vi "SP_OEE_2_test.vi"() -> ()   [LabVIEW 2017] (continued)
                      tunnel: [w1109] -> w922
                      tunnel: w1000 -> [w1148]
                      tunnel: w999 -> [w1147]
                      tunnel: w998 -> [w1146]
                      tunnel: w997 -> [w1142]
                      tunnel: w996 -> [w1145]
                      tunnel: w995 -> [w1144]
                      tunnel: w994 -> [w1140]
                      tunnel: w993 -> [w1138]
                      tunnel: w992 -> [w1137]
                      tunnel: [w1148] -> w988
                      tunnel: [w1147] -> w987
                      tunnel: [w1146] -> w986
                      tunnel: [w1145] -> w985
                      tunnel: [w1144] -> w984
                      tunnel: [w1141] -> w983
                      tunnel: [w1135] -> w982
                      tunnel: [w1134] -> w981
                      tunnel: [w1139] -> w980
                      tunnel: [w1138] -> w979
                      tunnel: [w1137] -> w978
                      tunnel: w991 -> [w1133]
                      tunnel: [w1133] -> w977
                      tunnel: w990 -> [w1130]
                      tunnel: [w1130] -> w976
                      tunnel: [w1129] -> w975
                      tunnel: w989 -> [w1129]
                      tunnel: w922 -> [w1128]
                      tunnel: [w1128] -> w921
                      tunnel: w988 -> [w1171]
                      tunnel: w987 -> [w1170]
                      tunnel: w986 -> [w1169]
                      tunnel: w985 -> [w1168]
                      tunnel: w984 -> [w1167]
                      tunnel: w983 -> [w1163]
                      tunnel: w982 -> [w1166]
                      tunnel: w981 -> [w1165]
                      tunnel: w980 -> [w1162]
                      tunnel: w979 -> [w1159]
                      tunnel: w978 -> [w1158]
                      tunnel: [w1171] -> w974
                      tunnel: [w1170] -> w973
                      tunnel: [w1169] -> w972
                      tunnel: [w1168] -> w971
                      tunnel: [w1167] -> w970
                      tunnel: [w1166] -> w969
                      tunnel: [w1165] -> w968
                      tunnel: [w1161] -> w967
                      tunnel: [w1160] -> w966
                      tunnel: [w1156] -> w965
                      tunnel: [w1155] -> w964
                      tunnel: [w1159] -> w963
                      tunnel: [w1158] -> w962
                      tunnel: w977 -> [w1154]
                      tunnel: [w1154] -> w961
                      tunnel: w976 -> [w1151]
                      tunnel: [w1151] -> w960
                      tunnel: [w1150] -> w959
                      tunnel: w975 -> [w1150]
                      tunnel: w921 -> [w1149]
                      tunnel: [w1149] -> w920
                      tunnel: w974 -> [w1196]
                      tunnel: w973 -> [w1195]
                      tunnel: w972 -> [w1194]
                      tunnel: w971 -> [w1193]
                      tunnel: w970 -> [w1192]
                      tunnel: w969 -> [w1191]
                      tunnel: w968 -> [w1190]
                      tunnel: w967 -> [w1184]
                      tunnel: w966 -> [w1186]
                      tunnel: w965 -> [w1189]
                      tunnel: w964 -> [w1188]
                      tunnel: w963 -> [w1181]
                      tunnel: w962 -> [w1182]
                      tunnel: [w1196] -> w958
                      tunnel: [w1195] -> w957
                      tunnel: [w1194] -> w956
                      tunnel: [w1193] -> w955
                      tunnel: [w1192] -> w954
                      tunnel: [w1191] -> w953
                      tunnel: [w1190] -> w952
                      tunnel: [w1189] -> w951
                      tunnel: [w1188] -> w950
                      tunnel: [w1185] -> w949
                      tunnel: [w1183] -> w948
                      tunnel: [w1179] -> w947
                      tunnel: [w1177] -> w946
                      tunnel: w961 -> [w1178]
                      tunnel: w960 -> [w1174]
                      tunnel: [w1173] -> w945
                      tunnel: w959 -> [w1173]
                      tunnel: w920 -> [w1172]
                      tunnel: w958 -> [w1223]
                      tunnel: w957 -> [w1216]
                      tunnel: w956 -> [w1207]
                      tunnel: w955 -> [w1215]
                      tunnel: w954 -> [w1205]
                      tunnel: w953 -> [w1214]
                      tunnel: w952 -> [w1203]
                      tunnel: w951 -> [w1213]
                      tunnel: w950 -> [w1201]
                      tunnel: w949 -> [w1237]
                      tunnel: w948 -> [w1236]
                      tunnel: w947 -> [w1212]
                      tunnel: w946 -> [w1199]
                      tunnel: [w1237] -> w944
                      tunnel: [w1236] -> w943
                      tunnel: [w1230] -> w942
                      tunnel: [w1223] -> w941
                      tunnel: [w1222] -> w940
                      tunnel: [w1221] -> w939
                      tunnel: [w1220] -> w938
                      tunnel: [w1219] -> w937
                      tunnel: [w1218] -> w936
                      tunnel: [w1217] -> w935
                      tunnel: [w1216] -> w934
                      tunnel: [w1215] -> w933
                      tunnel: [w1214] -> w932
                      tunnel: [w1213] -> w931
                      tunnel: [w1212] -> w930
                      tunnel: [w1197] -> w929
                      tunnel: w945 -> [w1197]
                      tunnel: [w1257] -> w904
                      tunnel: [w1243] -> w902
                      tunnel: w944 -> [w1244]
                      tunnel: w943 -> [w1257]
                      tunnel: w942 -> [w1242]
                      tunnel: w941 -> [w1255]
                      tunnel: w940 -> [w1253]
                      tunnel: w939 -> [w1251]
                      tunnel: w938 -> [w1249]
                      tunnel: w937 -> [w1247]
                      tunnel: w936 -> [w1245]
                      tunnel: w935 -> [w1238]
                      tunnel: w934 -> [w1254]
                      tunnel: w933 -> [w1252]
                      tunnel: w932 -> [w1250]
                      tunnel: w931 -> [w1248]
                      tunnel: w930 -> [w1246]
                      tunnel: w929 -> [w1241]
                      tunnel: [w1238] -> w916
                      frame #0 {
                        w1033 = "%Y-%m-%d" ("time format string (%c)")
                        n185 = Decimal String To Number(string=w1020) -> (number=w1019:i32)  [unwired: 2 in, 1 out]
                        n186 = property on="Table" class="Tbl (strict)"("Visible"=TRUE) -> ()  [unwired: 2 in, 2 out]
                        n187 = Format Date/Time String(time format string (%c)=w1033, seconds (now)=w1025) -> (date/time string=w1034:string)  [unwired: 1 in]
                        n188 = Format Date/Time String(time format string (%c)=w1033, seconds (now)=w1024) -> (date/time string=w1032:string)  [unwired: 1 in]
                        n189 = Format Into String(format string="Where BREAKDOWN_DATE between '%s' and '%s' and  SHIFT_ID = '%d'  ", w1034, w1032, w1019) -> (resulting string=w1031:string)  [unwired: 2 in, 1 out]
                        n190 = call <vilib>:"DB Tools Select Data.vi"("condition"=w1031, "error in (no error)"=w1040, "columns"=string[] ["BREAKDOWN_DATE"], "table"="STATION_1_LOG_HISTORY", "connection reference"=w1042) -> ("error out"=w1027:errorcluster, "data"=w1030:variant[][], "connection reference out"=w1041:T2)  [unwired: 1 in]
                        n191 = property on="Table 2" class="Tbl (strict)"("Visible"=FALSE) -> ()  [unwired: 2 in, 2 out]
                        n192 = xnode "Database Variant To Data"("database variant"=w1030, "error in (no error)"=w1027, "type"=string[][] [] ("Elements Found")) -> ("data"=w1028:string[][], "error out"=w1026:errorcluster)
                        n193 = Index Array(array=w1028, index (col)=0 ("disabled index (col)")) -> (element=w1036:string[])  [unwired: 1 in]
                        n194 = call "Search_1d_array_element.vi"("Count in"=string[] [] ("Elements Found"), "BD Date"=w1036, "Elements Found in"=string[] [] ("Elements Found")) -> ("Elements Found out"=w1022:string[])  [unwired: 4 in, 2 out]
                        n195 = Build Array(w1022) -> (w1046:string[][])
                        n196 = Transpose 2D Array(2D array=w1046) -> (transposed array=w1045:string[][])
                      }
                      frame #1 {
                        n197 = call "Stack_holderwise_total_bd_count_&_duration_2.vi"("Refnum in"=w1108, "BREAKDOWN_STK_HOLD_ID"=1, "condition"=w1095, "Form Date"=w1102, "To Date"=w1101, "error in (no error)"=w1106, "Shift"=w1092) -> ("Refnum out"=w1107:T2, "Count out"=w1100:string[], "appended array"=w1097:dbl[], "error out"=w1105:errorcluster)  [unwired: 5 in]
                        n198 = call "NUMERIC TO STRING.vi"("appended array"=w1097) -> ("Array"=w1096:string[])  [unwired: 4 in]
                        n199 = call "Insert_empty_element_with_zero.vi"("searched date"=w1100, "fixed date"=w1098) -> ("O/P"=w1093:string[])  [unwired: 9 in]
                        n200 = call "Insert_empty_element_with_zero.vi"("searched date"=w1096, "fixed date"=w1098) -> ("O/P"=w1099:string[])  [unwired: 9 in]
                      }
                      frame #2 {
                        n201 = call "Stack_holderwise_total_bd_count_&_duration_2.vi"("Refnum in"=w1122, "BREAKDOWN_STK_HOLD_ID"=2, "condition"=w1111, "Form Date"=w1119, "To Date"=w1118, "error in (no error)"=w1124, "Shift"=w1109) -> ("Refnum out"=w1120:T2, "Count out"=w1117:string[], "appended array"=w1113:dbl[], "error out"=w1123:errorcluster)  [unwired: 5 in]
                        n202 = call "Insert_empty_element_with_zero.vi"("searched date"=w1117, "fixed date"=w1114) -> ("O/P"=w1116:string[])  [unwired: 9 in]
                        n203 = call "NUMERIC TO STRING.vi"("appended array"=w1113) -> ("Array"=w1112:string[])  [unwired: 4 in]
                        n204 = call "Insert_empty_element_with_zero.vi"("searched date"=w1112, "fixed date"=w1114) -> ("O/P"=w1115:string[])  [unwired: 9 in]
                      }
                      frame #3 {
                        n205 = call "Stack_holderwise_total_bd_count_&_duration_2.vi"("Refnum in"=w1140, "BREAKDOWN_STK_HOLD_ID"=3, "condition"=w1130, "Form Date"=w1138, "To Date"=w1137, "error in (no error)"=w1142, "Shift"=w1128) -> ("Refnum out"=w1139:T2, "Count out"=w1136:string[], "appended array"=w1132:dbl[], "error out"=w1141:errorcluster)  [unwired: 5 in]
                        n206 = call "Insert_empty_element_with_zero.vi"("searched date"=w1136, "fixed date"=w1133) -> ("O/P"=w1135:string[])  [unwired: 9 in]
                        n207 = call "NUMERIC TO STRING.vi"("appended array"=w1132) -> ("Array"=w1131:string[])  [unwired: 4 in]
                        n208 = call "Insert_empty_element_with_zero.vi"("searched date"=w1131, "fixed date"=w1133) -> ("O/P"=w1134:string[])  [unwired: 9 in]
                      }
                      frame #4 {
                        n209 = call "Stack_holderwise_total_bd_count_&_duration_2.vi"("Refnum in"=w1162, "BREAKDOWN_STK_HOLD_ID"=4, "condition"=w1151, "Form Date"=w1159, "To Date"=w1158, "error in (no error)"=w1163, "Shift"=w1149) -> ("Refnum out"=w1161:T2, "Count out"=w1157:string[], "appended array"=w1153:dbl[], "error out"=w1160:errorcluster)  [unwired: 5 in]
                        n210 = call "Insert_empty_element_with_zero.vi"("searched date"=w1157, "fixed date"=w1154) -> ("O/P"=w1156:string[])  [unwired: 9 in]
                        n211 = call "NUMERIC TO STRING.vi"("appended array"=w1153) -> ("Array"=w1152:string[])  [unwired: 4 in]
                        n212 = call "Insert_empty_element_with_zero.vi"("searched date"=w1152, "fixed date"=w1154) -> ("O/P"=w1155:string[])  [unwired: 9 in]
                      }
                      frame #5 {
                        n213 = call "Stack_holderwise_total_bd_count_&_duration_2.vi"("Refnum in"=w1184, "BREAKDOWN_STK_HOLD_ID"=5, "condition"=w1174, "Form Date"=w1181, "To Date"=w1182, "error in (no error)"=w1186, "Shift"=w1172) -> ("Refnum out"=w1183:T2, "Count out"=w1180:string[], "appended array"=w1176:dbl[], "error out"=w1185:errorcluster)  [unwired: 5 in]
                        n214 = call "NUMERIC TO STRING.vi"("appended array"=w1176) -> ("Array"=w1175:string[])  [unwired: 4 in]
                        n215 = call "Insert_empty_element_with_zero.vi"("searched date"=w1180, "fixed date"=w1178) -> ("O/P"=w1179:string[])  [unwired: 9 in]
                        n216 = call "Insert_empty_element_with_zero.vi"("searched date"=w1175, "fixed date"=w1178) -> ("O/P"=w1177:string[])  [unwired: 9 in]
                      }
                      frame #6 {
                        n217 = call "String to numeric.vi"("Array"=w1207) -> ("Array 2"=w1206:dbl[])  [unwired: 4 in]
                        n218 = call "String to numeric.vi"("Array"=w1205) -> ("Array 2"=w1204:dbl[])  [unwired: 4 in]
                        n219 = call "String to numeric.vi"("Array"=w1203) -> ("Array 2"=w1202:dbl[])  [unwired: 4 in]
                        n220 = call "String to numeric.vi"("Array"=w1201) -> ("Array 2"=w1200:dbl[])  [unwired: 4 in]
                        n221 = call "String to numeric.vi"("Array"=w1199) -> ("Array 2"=w1198:dbl[])  [unwired: 4 in]
                        n222 = Decimal String To Number(string=w1212) -> (number=w1231:i32[])  [unwired: 2 in, 1 out]
                        n223 = Decimal String To Number(string=w1213) -> (number=w1232:i32[])  [unwired: 2 in, 1 out]
                        n224 = Decimal String To Number(string=w1214) -> (number=w1233:i32[])  [unwired: 2 in, 1 out]
                        n225 = Decimal String To Number(string=w1215) -> (number=w1234:i32[])  [unwired: 2 in, 1 out]
                        n226 = Decimal String To Number(string=w1216) -> (number=w1229:i32[])  [unwired: 2 in, 1 out]
                        n227 = Compound Arithmetic op=ADD(w1206, w1204, w1202, w1200, w1198) -> (w1209:dbl[])
                        n228 = Build Array(w1207) -> (w1228:string[][])
                        n229 = Build Array(w1205) -> (w1227:string[][])
                        n230 = Build Array(w1203) -> (w1226:string[][])
                        n231 = Build Array(w1201) -> (w1225:string[][])
                        n232 = Build Array(w1199) -> (w1224:string[][])
                        n233 = Number To Fractional String(number=w1209, precision (6)=i16 2) -> (F-format string=w1208:string[])  [unwired: 2 in]
                        n234 = Compound Arithmetic op=ADD(w1231, w1232, w1233, w1234, w1229) -> (w1235:i32[])
                        n235 = Transpose 2D Array(2D array=w1228) -> (transposed array=w1222:string[][])
                        n236 = Transpose 2D Array(2D array=w1227) -> (transposed array=w1221:string[][])
                        n237 = Transpose 2D Array(2D array=w1226) -> (transposed array=w1220:string[][])
                        n238 = Transpose 2D Array(2D array=w1225) -> (transposed array=w1219:string[][])
                        n239 = Transpose 2D Array(2D array=w1224) -> (transposed array=w1218:string[][])
                        n240 = Number To Decimal String(number=w1235) -> (decimal integer string=w1230:string[])  [unwired: 1 in]
                        n241 = Build Array(w1208) -> (w1211:string[][])
                        n242 = Transpose 2D Array(2D array=w1211) -> (transposed array=w1217:string[][])
                      }
                      frame #7 {
                        n243 = Insert Into Array(array=w1255, index (col)=1 ("disabled index (col)"), new element #1=w1254, new element #2=w1253, new element #3=w1252, new element #4=w1251, new element #5=w1250, new element #6=w1249, new element #7=w1248, new element #8=w1247, new element #9=w1246, new element #10=w1245, new element #11=w1242, new element #12=w1238) -> (w1240:string[][])  [unwired: 1 in]
                        n244 = call "flot graph for month n year.vi"("BD Date"=w1241, "error in (no error)"=w1244, "Count total"=w1242) -> ("error out"=w1243:errorcluster, "Run-Time Status"=w1239:cluster{"Array 2":timestamp[], dbl[]})  [unwired: 7 in]
                        n245 = local write "Run-Time Status"(w1239) -> ()
                        n246 = local write "Table"(w1240) -> ()
                      }
                    }
                    n247 = call "OEE_PART_1.vi"("CYCLE TIME"=w917, "ACTUAL PROD TIME"=w918, "BREAKDOWN TOTAL TIME"=w916) -> ("Numeric"=w907:i32, "CAPACITY"=w905:dbl, "ACTUAL TIME"=w906:i32)  [unwired: 5 in, 1 out]
                    n248 = call "OEE_PART_2_P.vi"("Refnum in"=w904, "Shift"=w913, "String"="ALL", "Select Station"=w911, "Form Date"=w915, "To Date"=w914, "AVAILABLILITY TIME"=w906, "CAPACITY"=w905) -> ("Refnum out"=w903:T2, "QUALITY"=w910:dbl, "OEE"=w908:dbl, "PERFORMANCE"=w909:dbl)  [unwired: 2 in, 2 out]
                    n249 = local write "PERFORMANCE"(w909) -> ()
                    n250 = local write "QUALITY"(w910) -> ()
                    n251 = local write "OEE"(w908) -> ()
                    n252 = local write "AVAILABLILITY TIME(MIN)"(w906) -> ()
                    n253 = local write "IDEAL CYCLE TIME"(w907) -> ()
                    n254 = local write "CAPACITY"(w905) -> ()
                  }
                  frame "3" {
                    n255 = flat-sequence {
                      tunnel: w1284 -> [w1398]
                      tunnel: w1283 -> [w1396]
                      tunnel: [w1382] -> w1374
                      tunnel: [w1397] -> w1373
                      tunnel: w1282 -> [_]
                      tunnel: [w1401] -> w1372
                      tunnel: [w1381] -> w1371
                      tunnel: [w1380] -> w1370
                      tunnel: [w1378] -> w1369
                      tunnel: w1281 -> [w1381]
                      tunnel: w1280 -> [w1380]
                      tunnel: ["Where BREAKDOWN_DATE between '%s'and '%s' and BREAKDOWN_STK_HOLD_ID ='%d' and  SHIFT_ID = '%d' "] -> w1368
                      tunnel: [w1378] -> w1367
                      tunnel: w1275 -> [w1376]
                      tunnel: w1374 -> [w1462]
                      tunnel: w1373 -> [w1464]
                      tunnel: w1372 -> [w1459]
                      tunnel: w1371 -> [w1458]
                      tunnel: w1370 -> [w1457]
                      tunnel: [w1461] -> w1366
                      tunnel: [w1463] -> w1365
                      tunnel: [w1459] -> w1364
                      tunnel: [w1449] -> w1363
                      tunnel: [w1455] -> w1362
                      tunnel: [w1458] -> w1361
                      tunnel: [w1457] -> w1360
                      tunnel: w1369 -> [w1454]
                      tunnel: [w1454] -> w1359
                      tunnel: w1368 -> [w1451]
                      tunnel: [w1451] -> w1358
                      tunnel: [w1450] -> w1357
                      tunnel: w1367 -> [w1450]
                      tunnel: w1275 -> [w1448]
                      tunnel: [w1448] -> w1279
                      tunnel: w1366 -> [w1480]
                      tunnel: w1365 -> [w1478]
                      tunnel: w1364 -> [w1483]
                      tunnel: w1363 -> [w1482]
                      tunnel: w1362 -> [w1481]
                      tunnel: w1361 -> [w1475]
                      tunnel: w1360 -> [w1474]
                      tunnel: [w1483] -> w1356
                      tunnel: [w1482] -> w1355
                      tunnel: [w1481] -> w1354
                      tunnel: [w1479] -> w1353
                      tunnel: [w1472] -> w1352
                      tunnel: [w1471] -> w1351
                      tunnel: [w1476] -> w1350
                      tunnel: [w1475] -> w1349
                      tunnel: [w1474] -> w1348
                      tunnel: w1359 -> [w1470]
                      tunnel: [w1470] -> w1347
                      tunnel: w1358 -> [w1467]
                      tunnel: [w1467] -> w1346
                      tunnel: [w1466] -> w1345
                      tunnel: w1357 -> [w1466]
                      tunnel: w1279 -> [w1465]
                      tunnel: [w1465] -> w1278
                      tunnel: w1356 -> [w1504]
                      tunnel: w1355 -> [w1503]
                      tunnel: w1354 -> [w1502]
                      tunnel: w1353 -> [w1498]
                      tunnel: w1352 -> [w1501]
                      tunnel: w1351 -> [w1500]
                      tunnel: w1350 -> [w1496]
                      tunnel: w1349 -> [w1494]
                      tunnel: w1348 -> [w1493]
                      tunnel: [w1504] -> w1344
                      tunnel: [w1503] -> w1343
                      tunnel: [w1502] -> w1342
                      tunnel: [w1501] -> w1341
                      tunnel: [w1500] -> w1340
                      tunnel: [w1497] -> w1339
                      tunnel: [w1491] -> w1338
                      tunnel: [w1490] -> w1337
                      tunnel: [w1495] -> w1336
                      tunnel: [w1494] -> w1335
                      tunnel: [w1493] -> w1334
                      tunnel: w1347 -> [w1489]
                      tunnel: [w1489] -> w1333
                      tunnel: w1346 -> [w1486]
                      tunnel: [w1486] -> w1332
                      tunnel: [w1485] -> w1331
                      tunnel: w1345 -> [w1485]
                      tunnel: w1278 -> [w1484]
                      tunnel: [w1484] -> w1277
                      tunnel: w1344 -> [w1527]
                      tunnel: w1343 -> [w1526]
                      tunnel: w1342 -> [w1525]
                      tunnel: w1341 -> [w1524]
                      tunnel: w1340 -> [w1523]
                      tunnel: w1339 -> [w1519]
                      tunnel: w1338 -> [w1522]
                      tunnel: w1337 -> [w1521]
                      tunnel: w1336 -> [w1518]
                      tunnel: w1335 -> [w1515]
                      tunnel: w1334 -> [w1514]
                      tunnel: [w1527] -> w1330
                      tunnel: [w1526] -> w1329
                      tunnel: [w1525] -> w1328
                      tunnel: [w1524] -> w1327
                      tunnel: [w1523] -> w1326
                      tunnel: [w1522] -> w1325
                      tunnel: [w1521] -> w1324
                      tunnel: [w1517] -> w1323
                      tunnel: [w1516] -> w1322
                      tunnel: [w1512] -> w1321
                      tunnel: [w1511] -> w1320
                      tunnel: [w1515] -> w1319
                      tunnel: [w1514] -> w1318
                      tunnel: w1333 -> [w1510]
                      tunnel: [w1510] -> w1317
                      tunnel: w1332 -> [w1507]
                      tunnel: [w1507] -> w1316
                      tunnel: [w1506] -> w1315
                      tunnel: w1331 -> [w1506]
                      tunnel: w1277 -> [w1505]
                      tunnel: [w1505] -> w1276
                      tunnel: w1330 -> [w1552]
                      tunnel: w1329 -> [w1551]
                      tunnel: w1328 -> [w1550]
                      tunnel: w1327 -> [w1549]
                      tunnel: w1326 -> [w1548]
                      tunnel: w1325 -> [w1547]
                      tunnel: w1324 -> [w1546]
                      tunnel: w1323 -> [w1540]
                      tunnel: w1322 -> [w1542]
                      tunnel: w1321 -> [w1545]
                      tunnel: w1320 -> [w1544]
                      tunnel: w1319 -> [w1537]
                      tunnel: w1318 -> [w1538]
                      tunnel: [w1552] -> w1314
                      tunnel: [w1551] -> w1313
                      tunnel: [w1550] -> w1312
                      tunnel: [w1549] -> w1311
                      tunnel: [w1548] -> w1310
                      tunnel: [w1547] -> w1309
                      tunnel: [w1546] -> w1308
                      tunnel: [w1545] -> w1307
                      tunnel: [w1544] -> w1306
                      tunnel: [w1541] -> w1305
                      tunnel: [w1539] -> w1304
                      tunnel: [w1535] -> w1303
                      tunnel: [w1533] -> w1302
                      tunnel: w1317 -> [w1534]
                      tunnel: w1316 -> [w1530]
                      tunnel: [w1529] -> w1301
                      tunnel: w1315 -> [w1529]
                      tunnel: w1276 -> [w1528]
                      tunnel: w1314 -> [w1579]
                      tunnel: w1313 -> [w1572]
                      tunnel: w1312 -> [w1563]
                      tunnel: w1311 -> [w1571]
                      tunnel: w1310 -> [w1561]
                      tunnel: w1309 -> [w1570]
                      tunnel: w1308 -> [w1559]
                      tunnel: w1307 -> [w1569]
                      tunnel: w1306 -> [w1557]
                      tunnel: w1305 -> [w1593]
                      tunnel: w1304 -> [w1592]
                      tunnel: w1303 -> [w1568]
                      tunnel: w1302 -> [w1555]
                      tunnel: [w1593] -> w1300
                      tunnel: [w1592] -> w1299
                      tunnel: [w1586] -> w1298
                      tunnel: [w1579] -> w1297
                      tunnel: [w1578] -> w1296
                      tunnel: [w1577] -> w1295
                      tunnel: [w1576] -> w1294
                      tunnel: [w1575] -> w1293
                      tunnel: [w1574] -> w1292
                      tunnel: [w1573] -> w1291
                      tunnel: [w1572] -> w1290
                      tunnel: [w1571] -> w1289
                      tunnel: [w1570] -> w1288
                      tunnel: [w1569] -> w1287
                      tunnel: [w1568] -> w1286
                      tunnel: [w1553] -> w1285
                      tunnel: w1301 -> [w1553]
                      tunnel: [w1613] -> w1260
                      tunnel: [w1599] -> w1258
                      tunnel: w1300 -> [w1600]
                      tunnel: w1299 -> [w1613]
                      tunnel: w1298 -> [w1598]
                      tunnel: w1297 -> [w1611]
                      tunnel: w1296 -> [w1609]
                      tunnel: w1295 -> [w1607]
                      tunnel: w1294 -> [w1605]
                      tunnel: w1293 -> [w1603]
                      tunnel: w1292 -> [w1601]
                      tunnel: w1291 -> [w1594]
                      tunnel: w1290 -> [w1610]
                      tunnel: w1289 -> [w1608]
                      tunnel: w1288 -> [w1606]
                      tunnel: w1287 -> [w1604]
                      tunnel: w1286 -> [w1602]
                      tunnel: w1285 -> [w1597]
                      tunnel: [w1594] -> w1271
                      frame #0 {
                        w1389 = "%Y-%m-%d" ("time format string (%c)")
                        n256 = Decimal String To Number(string=w1376) -> (number=w1375:i32)  [unwired: 2 in, 1 out]
                        n257 = property on="Table" class="Tbl (strict)"("Visible"=TRUE) -> ()  [unwired: 2 in, 2 out]
                        n258 = Format Date/Time String(time format string (%c)=w1389, seconds (now)=w1381) -> (date/time string=w1390:string)  [unwired: 1 in]
                        n259 = Format Date/Time String(time format string (%c)=w1389, seconds (now)=w1380) -> (date/time string=w1388:string)  [unwired: 1 in]
                        n260 = Format Into String(format string="Where BREAKDOWN_DATE between '%s' and '%s' and  SHIFT_ID = '%d'  ", w1390, w1388, w1375) -> (resulting string=w1387:string)  [unwired: 2 in, 1 out]
                        n261 = call <vilib>:"DB Tools Select Data.vi"("condition"=w1387, "error in (no error)"=w1396, "columns"=string[] ["BREAKDOWN_DATE"], "table"="STATION_1_LOG_HISTORY", "connection reference"=w1398) -> ("error out"=w1383:errorcluster, "data"=w1386:variant[][], "connection reference out"=w1397:T2)  [unwired: 1 in]
                        n262 = property on="Table 2" class="Tbl (strict)"("Visible"=FALSE) -> ()  [unwired: 2 in, 2 out]
                        n263 = xnode "Database Variant To Data"("database variant"=w1386, "error in (no error)"=w1383, "type"=string[][] [] ("Elements Found")) -> ("data"=w1384:string[][], "error out"=w1382:errorcluster)
                        n264 = Index Array(array=w1384, index (col)=0 ("disabled index (col)")) -> (element=w1392:string[])  [unwired: 1 in]
                        n265 = call "Search_1d_array_element.vi"("Count in"=string[] [] ("Elements Found"), "BD Date"=w1392, "Elements Found in"=string[] [] ("Elements Found")) -> ("Elements Found out"=w1378:string[])  [unwired: 4 in, 2 out]
                        n266 = Build Array(w1378) -> (w1402:string[][])
                        n267 = Transpose 2D Array(2D array=w1402) -> (transposed array=w1401:string[][])
                      }
                      frame #1 {
                        n268 = call "Stack_holderwise_total_bd_count_&_duration_2.vi"("Refnum in"=w1464, "BREAKDOWN_STK_HOLD_ID"=1, "condition"=w1451, "Form Date"=w1458, "To Date"=w1457, "error in (no error)"=w1462, "Shift"=w1448) -> ("Refnum out"=w1463:T2, "Count out"=w1456:string[], "appended array"=w1453:dbl[], "error out"=w1461:errorcluster)  [unwired: 5 in]
                        n269 = call "NUMERIC TO STRING.vi"("appended array"=w1453) -> ("Array"=w1452:string[])  [unwired: 4 in]
                        n270 = call "Insert_empty_element_with_zero.vi"("searched date"=w1456, "fixed date"=w1454) -> ("O/P"=w1449:string[])  [unwired: 9 in]
                        n271 = call "Insert_empty_element_with_zero.vi"("searched date"=w1452, "fixed date"=w1454) -> ("O/P"=w1455:string[])  [unwired: 9 in]
                      }
                      frame #2 {
                        n272 = call "Stack_holderwise_total_bd_count_&_duration_2.vi"("Refnum in"=w1478, "BREAKDOWN_STK_HOLD_ID"=2, "condition"=w1467, "Form Date"=w1475, "To Date"=w1474, "error in (no error)"=w1480, "Shift"=w1465) -> ("Refnum out"=w1476:T2, "Count out"=w1473:string[], "appended array"=w1469:dbl[], "error out"=w1479:errorcluster)  [unwired: 5 in]
                        n273 = call "Insert_empty_element_with_zero.vi"("searched date"=w1473, "fixed date"=w1470) -> ("O/P"=w1472:string[])  [unwired: 9 in]
                        n274 = call "NUMERIC TO STRING.vi"("appended array"=w1469) -> ("Array"=w1468:string[])  [unwired: 4 in]
                        n275 = call "Insert_empty_element_with_zero.vi"("searched date"=w1468, "fixed date"=w1470) -> ("O/P"=w1471:string[])  [unwired: 9 in]
                      }
                      frame #3 {
                        n276 = call "Stack_holderwise_total_bd_count_&_duration_2.vi"("Refnum in"=w1496, "BREAKDOWN_STK_HOLD_ID"=3, "condition"=w1486, "Form Date"=w1494, "To Date"=w1493, "error in (no error)"=w1498, "Shift"=w1484) -> ("Refnum out"=w1495:T2, "Count out"=w1492:string[], "appended array"=w1488:dbl[], "error out"=w1497:errorcluster)  [unwired: 5 in]
                        n277 = call "Insert_empty_element_with_zero.vi"("searched date"=w1492, "fixed date"=w1489) -> ("O/P"=w1491:string[])  [unwired: 9 in]
                        n278 = call "NUMERIC TO STRING.vi"("appended array"=w1488) -> ("Array"=w1487:string[])  [unwired: 4 in]
                        n279 = call "Insert_empty_element_with_zero.vi"("searched date"=w1487, "fixed date"=w1489) -> ("O/P"=w1490:string[])  [unwired: 9 in]
                      }
                      frame #4 {
                        n280 = call "Stack_holderwise_total_bd_count_&_duration_2.vi"("Refnum in"=w1518, "BREAKDOWN_STK_HOLD_ID"=4, "condition"=w1507, "Form Date"=w1515, "To Date"=w1514, "error in (no error)"=w1519, "Shift"=w1505) -> ("Refnum out"=w1517:T2, "Count out"=w1513:string[], "appended array"=w1509:dbl[], "error out"=w1516:errorcluster)  [unwired: 5 in]
                        n281 = call "Insert_empty_element_with_zero.vi"("searched date"=w1513, "fixed date"=w1510) -> ("O/P"=w1512:string[])  [unwired: 9 in]
                        n282 = call "NUMERIC TO STRING.vi"("appended array"=w1509) -> ("Array"=w1508:string[])  [unwired: 4 in]
                        n283 = call "Insert_empty_element_with_zero.vi"("searched date"=w1508, "fixed date"=w1510) -> ("O/P"=w1511:string[])  [unwired: 9 in]
                      }
                      frame #5 {
                        n284 = call "Stack_holderwise_total_bd_count_&_duration_2.vi"("Refnum in"=w1540, "BREAKDOWN_STK_HOLD_ID"=5, "condition"=w1530, "Form Date"=w1537, "To Date"=w1538, "error in (no error)"=w1542, "Shift"=w1528) -> ("Refnum out"=w1539:T2, "Count out"=w1536:string[], "appended array"=w1532:dbl[], "error out"=w1541:errorcluster)  [unwired: 5 in]
                        n285 = call "NUMERIC TO STRING.vi"("appended array"=w1532) -> ("Array"=w1531:string[])  [unwired: 4 in]
                        n286 = call "Insert_empty_element_with_zero.vi"("searched date"=w1536, "fixed date"=w1534) -> ("O/P"=w1535:string[])  [unwired: 9 in]
                        n287 = call "Insert_empty_element_with_zero.vi"("searched date"=w1531, "fixed date"=w1534) -> ("O/P"=w1533:string[])  [unwired: 9 in]
                      }
                      frame #6 {
                        n288 = call "String to numeric.vi"("Array"=w1563) -> ("Array 2"=w1562:dbl[])  [unwired: 4 in]
                        n289 = call "String to numeric.vi"("Array"=w1561) -> ("Array 2"=w1560:dbl[])  [unwired: 4 in]
                        n290 = call "String to numeric.vi"("Array"=w1559) -> ("Array 2"=w1558:dbl[])  [unwired: 4 in]
                        n291 = call "String to numeric.vi"("Array"=w1557) -> ("Array 2"=w1556:dbl[])  [unwired: 4 in]
                        n292 = call "String to numeric.vi"("Array"=w1555) -> ("Array 2"=w1554:dbl[])  [unwired: 4 in]
                        n293 = Decimal String To Number(string=w1568) -> (number=w1587:i32[])  [unwired: 2 in, 1 out]
                        n294 = Decimal String To Number(string=w1569) -> (number=w1588:i32[])  [unwired: 2 in, 1 out]
                        n295 = Decimal String To Number(string=w1570) -> (number=w1589:i32[])  [unwired: 2 in, 1 out]
                        n296 = Decimal String To Number(string=w1571) -> (number=w1590:i32[])  [unwired: 2 in, 1 out]
                        n297 = Decimal String To Number(string=w1572) -> (number=w1585:i32[])  [unwired: 2 in, 1 out]
                        n298 = Compound Arithmetic op=ADD(w1562, w1560, w1558, w1556, w1554) -> (w1565:dbl[])
                        n299 = Build Array(w1563) -> (w1584:string[][])
                        n300 = Build Array(w1561) -> (w1583:string[][])
                        n301 = Build Array(w1559) -> (w1582:string[][])
                        n302 = Build Array(w1557) -> (w1581:string[][])
                        n303 = Build Array(w1555) -> (w1580:string[][])
                        n304 = Number To Fractional String(number=w1565, precision (6)=i16 2) -> (F-format string=w1564:string[])  [unwired: 2 in]
                        n305 = Compound Arithmetic op=ADD(w1587, w1588, w1589, w1590, w1585) -> (w1591:i32[])
                        n306 = Transpose 2D Array(2D array=w1584) -> (transposed array=w1578:string[][])
                        n307 = Transpose 2D Array(2D array=w1583) -> (transposed array=w1577:string[][])
                        n308 = Transpose 2D Array(2D array=w1582) -> (transposed array=w1576:string[][])
                        n309 = Transpose 2D Array(2D array=w1581) -> (transposed array=w1575:string[][])
                        n310 = Transpose 2D Array(2D array=w1580) -> (transposed array=w1574:string[][])
                        n311 = Number To Decimal String(number=w1591) -> (decimal integer string=w1586:string[])  [unwired: 1 in]
                        n312 = Build Array(w1564) -> (w1567:string[][])
                        n313 = Transpose 2D Array(2D array=w1567) -> (transposed array=w1573:string[][])
                      }
                      frame #7 {
                        n314 = Insert Into Array(array=w1611, index (col)=1 ("disabled index (col)"), new element #1=w1610, new element #2=w1609, new element #3=w1608, new element #4=w1607, new element #5=w1606, new element #6=w1605, new element #7=w1604, new element #8=w1603, new element #9=w1602, new element #10=w1601, new element #11=w1598, new element #12=w1594) -> (w1596:string[][])  [unwired: 1 in]
                        n315 = call "flot graph for month n year.vi"("BD Date"=w1597, "error in (no error)"=w1600, "Count total"=w1598) -> ("error out"=w1599:errorcluster, "Run-Time Status"=w1595:cluster{"Array 2":timestamp[], dbl[]})  [unwired: 7 in]
                        n316 = local write "Run-Time Status"(w1595) -> ()
                        n317 = local write "Table"(w1596) -> ()
                      }
                    }
                    n318 = call "OEE_PART_1.vi"("CYCLE TIME"=w1272, "ACTUAL PROD TIME"=w1273, "BREAKDOWN TOTAL TIME"=w1271) -> ("Numeric"=w1262:i32, "CAPACITY"=w1261:dbl, "ACTUAL TIME"=w1263:i32)  [unwired: 5 in, 1 out]
                    n319 = call "OEE_PART_2_P.vi"("Refnum in"=w1260, "Shift"=w1267, "String"="ALL", "Select Station"=w1268, "Form Date"=w1270, "To Date"=w1269, "AVAILABLILITY TIME"=w1263, "CAPACITY"=w1261) -> ("Refnum out"=w1259:T2, "QUALITY"=w1266:dbl, "OEE"=w1264:dbl, "PERFORMANCE"=w1265:dbl)  [unwired: 2 in, 2 out]
                    n320 = local write "PERFORMANCE"(w1265) -> ()
                    n321 = local write "QUALITY"(w1266) -> ()
                    n322 = local write "OEE"(w1264) -> ()
                    n323 = local write "AVAILABLILITY TIME(MIN)"(w1263) -> ()
                    n324 = local write "IDEAL CYCLE TIME"(w1262) -> ()
                    n325 = local write "CAPACITY"(w1261) -> ()
                  }
                  frame "all" {
                  }
                }
              }
              frame "Safety" {
                n326 = local read "Shift"() -> (w1616:string)
                n327 = case shown="\"1\"" w1616 {
                  selector: w1616 -> [_ w1991 w2362 w2731]
                  tunnel: w1621 -> [w1628 w1996 w2367 w2736]
                  tunnel: w1620 -> [w1627 w1995 w2366 w2735]
                  tunnel: w1619 -> [w1626 w1994 w2365 w2734]
                  tunnel: w1618 -> [w1625 w1993 w2364 w2733]
                  tunnel: w1617 -> [w1624 w1992 w2363 w2732]
                  tunnel: [w1623 w1989 w2360 _] -> w1615
                  tunnel: [w1622 w1988 w2359 _] -> w1614
                  frame "ALL", Default {
                    n328 = flat-sequence {
                      tunnel: w1628 -> [w1740]
                      tunnel: w1627 -> [w1738]
                      tunnel: [w1724] -> w1718
                      tunnel: [w1739] -> w1717
                      tunnel: w1626 -> [_]
                      tunnel: [w1743] -> w1716
                      tunnel: [w1723] -> w1715
                      tunnel: [w1722] -> w1714
                      tunnel: [w1720] -> w1713
                      tunnel: w1625 -> [w1723]
                      tunnel: w1624 -> [w1722]
                      tunnel: ["Where BREAKDOWN_DATE between '%s'and '%s' and BREAKDOWN_STK_HOLD_ID ='%d'  "] -> w1712
                      tunnel: [w1720] -> w1711
                      tunnel: w1718 -> [w1803]
                      tunnel: w1717 -> [w1805]
                      tunnel: w1716 -> [w1800]
                      tunnel: w1715 -> [w1799]
                      tunnel: w1714 -> [w1798]
                      tunnel: [w1802] -> w1710
                      tunnel: [w1804] -> w1709
                      tunnel: [w1800] -> w1708
                      tunnel: [w1790] -> w1707
                      tunnel: [w1796] -> w1706
                      tunnel: [w1799] -> w1705
                      tunnel: [w1798] -> w1704
                      tunnel: w1713 -> [w1795]
                      tunnel: [w1795] -> w1703
                      tunnel: w1712 -> [w1792]
                      tunnel: [w1792] -> w1702
                      tunnel: [w1791] -> w1701
                      tunnel: w1711 -> [w1791]
                      tunnel: w1710 -> [w1819]
                      tunnel: w1709 -> [w1817]
                      tunnel: w1708 -> [w1822]
                      tunnel: w1707 -> [w1821]
                      tunnel: w1706 -> [w1820]
                      tunnel: w1705 -> [w1815]
                      tunnel: w1704 -> [w1814]
                      tunnel: [w1822] -> w1700
                      tunnel: [w1821] -> w1699
                      tunnel: [w1820] -> w1698
                      tunnel: [w1818] -> w1697
                      tunnel: [w1812] -> w1696
                      tunnel: [w1811] -> w1695
                      tunnel: [w1816] -> w1694
                      tunnel: [w1815] -> w1693
                      tunnel: [w1814] -> w1692
                      tunnel: w1703 -> [w1810]
                      tunnel: [w1810] -> w1691
                      tunnel: w1702 -> [w1807]
                      tunnel: [w1807] -> w1690
                      tunnel: [w1806] -> w1689
                      tunnel: w1701 -> [w1806]
                      tunnel: w1700 -> [w1853]
                      tunnel: w1699 -> [w1852]
                      tunnel: w1698 -> [w1851]
                      tunnel: w1697 -> [w1848]
                      tunnel: w1696 -> [w1850]
                      tunnel: w1695 -> [w1849]
                      tunnel: w1694 -> [w1846]
                      tunnel: w1693 -> [w1844]
                      tunnel: w1692 -> [w1843]
                      tunnel: [w1853] -> w1688
                      tunnel: [w1852] -> w1687
                      tunnel: [w1851] -> w1686
                      tunnel: [w1850] -> w1685
                      tunnel: [w1849] -> w1684
                      tunnel: [w1847] -> w1683
                      tunnel: [w1841] -> w1682
                      tunnel: [w1840] -> w1681
                      tunnel: [w1845] -> w1680
                      tunnel: [w1844] -> w1679
                      tunnel: [w1843] -> w1678
                      tunnel: w1691 -> [w1839]
                      tunnel: [w1839] -> w1677
                      tunnel: w1690 -> [w1836]
                      tunnel: [w1836] -> w1676
                      tunnel: [w1835] -> w1675
                      tunnel: w1689 -> [w1835]
                      tunnel: w1688 -> [w1886]
                      tunnel: w1687 -> [w1885]
                      tunnel: w1686 -> [w1884]
                      tunnel: w1685 -> [w1883]
                      tunnel: w1684 -> [w1882]
                      tunnel: w1683 -> [w1879]
                      tunnel: w1682 -> [w1881]
                      tunnel: w1681 -> [w1880]
                      tunnel: w1680 -> [w1878]
                      tunnel: w1679 -> [w1875]
                      tunnel: w1678 -> [w1874]
                      tunnel: [w1886] -> w1674
                      tunnel: [w1885] -> w1673
                      tunnel: [w1884] -> w1672
                      tunnel: [w1883] -> w1671
                      tunnel: [w1882] -> w1670
                      tunnel: [w1881] -> w1669
                      tunnel: [w1880] -> w1668
                      tunnel: [w1877] -> w1667
                      tunnel: [w1876] -> w1666
                      tunnel: [w1872] -> w1665
                      tunnel: [w1871] -> w1664
                      tunnel: [w1875] -> w1663
                      tunnel: [w1874] -> w1662
                      tunnel: w1677 -> [w1870]
                      tunnel: [w1870] -> w1661
                      tunnel: w1676 -> [w1867]
                      tunnel: [w1867] -> w1660
                      tunnel: [w1866] -> w1659
                      tunnel: w1675 -> [w1866]
                      tunnel: w1674 -> [w1921]
                      tunnel: w1673 -> [w1920]
                      tunnel: w1672 -> [w1919]
                      tunnel: w1671 -> [w1918]
                      tunnel: w1670 -> [w1917]
                      tunnel: w1669 -> [w1916]
                      tunnel: w1668 -> [w1915]
                      tunnel: w1667 -> [w1910]
                      tunnel: w1666 -> [w1912]
                      tunnel: w1665 -> [w1914]
                      tunnel: w1664 -> [w1913]
                      tunnel: w1663 -> [w1907]
                      tunnel: w1662 -> [w1908]
                      tunnel: [w1921] -> w1658
                      tunnel: [w1920] -> w1657
                      tunnel: [w1919] -> w1656
                      tunnel: [w1918] -> w1655
                      tunnel: [w1917] -> w1654
                      tunnel: [w1916] -> w1653
                      tunnel: [w1915] -> w1652
                      tunnel: [w1914] -> w1651
                      tunnel: [w1913] -> w1650
                      tunnel: [w1911] -> w1649
                      tunnel: [w1909] -> w1648
                      tunnel: [w1905] -> w1647
                      tunnel: [w1903] -> w1646
                      tunnel: w1661 -> [w1904]
                      tunnel: w1660 -> [w1900]
                      tunnel: [w1899] -> w1645
                      tunnel: w1659 -> [w1899]
                      tunnel: w1658 -> [w1960]
                      tunnel: w1657 -> [w1953]
                      tunnel: w1656 -> [w1944]
                      tunnel: w1655 -> [w1952]
                      tunnel: w1654 -> [w1942]
                      tunnel: w1653 -> [w1951]
                      tunnel: w1652 -> [w1940]
                      tunnel: w1651 -> [w1950]
                      tunnel: w1650 -> [w1938]
                      tunnel: w1649 -> [w1974]
                      tunnel: w1648 -> [w1973]
                      tunnel: w1647 -> [w1949]
                      tunnel: w1646 -> [w1936]
                      tunnel: [w1974] -> w1644
                      tunnel: [w1973] -> w1643
                      tunnel: [w1967] -> w1642
                      tunnel: [w1960] -> w1641
                      tunnel: [w1959] -> w1640
                      tunnel: [w1958] -> w1639
                      tunnel: [w1957] -> w1638
                      tunnel: [w1956] -> w1637
                      tunnel: [w1955] -> w1636
                      tunnel: [w1954] -> w1635
                      tunnel: [w1953] -> w1634
                      tunnel: [w1952] -> w1633
                      tunnel: [w1951] -> w1632
                      tunnel: [w1950] -> w1631
                      tunnel: [w1949] -> w1630
                      tunnel: [w1934] -> w1629
                      tunnel: w1645 -> [w1934]
                      tunnel: [w1987] -> w1622
                      tunnel: [w1981] -> w1623
                      tunnel: w1644 -> [w1982]
                      tunnel: w1643 -> [w1987]
                      tunnel: w1642 -> [w1976]
                      tunnel: w1641 -> [w1985]
                      tunnel: w1640 -> [w1983]
                      tunnel: w1639 -> [_]
                      tunnel: w1638 -> [_]
                      tunnel: w1637 -> [_]
                      tunnel: w1636 -> [_]
                      tunnel: w1635 -> [w1977]
                      tunnel: w1634 -> [w1984]
                      tunnel: w1633 -> [_]
                      tunnel: w1632 -> [_]
                      tunnel: w1631 -> [_]
                      tunnel: w1630 -> [_]
                      tunnel: w1629 -> [w1980]
                      frame #0 {
                        w1731 = "%Y-%m-%d" ("time format string (%c)")
                        n329 = property on="Table" class="Tbl (strict)"("Visible"=TRUE) -> ()  [unwired: 2 in, 2 out]
                        n330 = Format Date/Time String(time format string (%c)=w1731, seconds (now)=w1723) -> (date/time string=w1732:string)  [unwired: 1 in]
                        n331 = Format Date/Time String(time format string (%c)=w1731, seconds (now)=w1722) -> (date/time string=w1730:string)  [unwired: 1 in]
                        n332 = Format Into String(format string="Where BREAKDOWN_DATE between '%s' and '%s' ", w1732, w1730) -> (resulting string=w1729:string)  [unwired: 2 in, 1 out]
                        n333 = call <vilib>:"DB Tools Select Data.vi"("condition"=w1729, "error in (no error)"=w1738, "columns"=string[] ["BREAKDOWN_DATE"], "table"="STATION_1_LOG_HISTORY", "connection reference"=w1740) -> ("error out"=w1725:errorcluster, "data"=w1728:variant[][], "connection reference out"=w1739:T2)  [unwired: 1 in]
                        n334 = property on="Table 2" class="Tbl (strict)"("Visible"=FALSE) -> ()  [unwired: 2 in, 2 out]
                        n335 = xnode "Database Variant To Data"("database variant"=w1728, "error in (no error)"=w1725, "type"=string[][] [] ("Elements Found")) -> ("data"=w1726:string[][], "error out"=w1724:errorcluster)
                        n336 = Index Array(array=w1726, index (col)=0 ("disabled index (col)")) -> (element=w1734:string[])  [unwired: 1 in]
                        n337 = call "Search_1d_array_element.vi"("Count in"=string[] [] ("Elements Found"), "BD Date"=w1734, "Elements Found in"=string[] [] ("Elements Found")) -> ("Elements Found out"=w1720:string[])  [unwired: 4 in, 2 out]
                        n338 = Build Array(w1720) -> (w1744:string[][])
                        n339 = Transpose 2D Array(2D array=w1744) -> (transposed array=w1743:string[][])
                      }
                      frame #1 {
                        n340 = call "Stack_holderwise_total_bd_count_&_duration.vi"("Refnum in"=w1805, "BREAKDOWN_STK_HOLD_ID"=1, "condition"=w1792, "Form Date"=w1799, "To Date"=w1798, "error in (no error)"=w1803) -> ("Refnum out"=w1804:T2, "Count out"=w1797:string[], "appended array"=w1794:dbl[], "error out"=w1802:errorcluster)  [unwired: 6 in]
                        n341 = call "NUMERIC TO STRING.vi"("appended array"=w1794) -> ("Array"=w1793:string[])  [unwired: 4 in]
                        n342 = call "Insert_empty_element_with_zero.vi"("searched date"=w1797, "fixed date"=w1795) -> ("O/P"=w1790:string[])  [unwired: 9 in]
                        n343 = call "Insert_empty_element_with_zero.vi"("searched date"=w1793, "fixed date"=w1795) -> ("O/P"=w1796:string[])  [unwired: 9 in]
                      }
                      frame #2 {
                        n344 = disable-structure shown="Enabled" {
                          disable-tunnel: w1819 -> [w1832 w1834]
                          disable-tunnel: [w1831 w1834] -> w1818
                          disable-tunnel: w1817 -> [w1830 w1833]
                          disable-tunnel: [w1828 w1833] -> w1816
                          disable-tunnel: w1815 -> [w1827 _]
                          disable-tunnel: w1814 -> [w1826 _]
                          disable-tunnel: [w1825 _] -> w1813
                          disable-tunnel: [w1824 _] -> w1809
                          disable-tunnel: w1807 -> [w1823 _]
                          frame Disabled {
                            n345 = call "Stack_holderwise_total_bd_count_&_duration.vi"("Refnum in"=w1830, "BREAKDOWN_STK_HOLD_ID"=2, "condition"=w1823, "Form Date"=w1827, "To Date"=w1826, "error in (no error)"=w1832) -> ("Refnum out"=w1828:T2, "Count out"=w1825:string[], "appended array"=w1824:dbl[], "error out"=w1831:errorcluster)  [unwired: 6 in]
                          }
                          frame Enabled {
                          }
                        }
                        n346 = call "Insert_empty_element_with_zero.vi"("searched date"=w1813, "fixed date"=w1810) -> ("O/P"=w1812:string[])  [unwired: 9 in]
                        n347 = call "NUMERIC TO STRING.vi"("appended array"=w1809) -> ("Array"=w1808:string[])  [unwired: 4 in]
                        n348 = call "Insert_empty_element_with_zero.vi"("searched date"=w1808, "fixed date"=w1810) -> ("O/P"=w1811:string[])  [unwired: 9 in]
                      }
                      frame #3 {
                        n349 = disable-structure shown="Enabled" {
                          disable-tunnel: w1848 -> [w1862 w1865]
                          disable-tunnel: [w1861 w1865] -> w1847
                          disable-tunnel: w1846 -> [w1860 w1864]
                          disable-tunnel: [w1859 w1864] -> w1845
                          disable-tunnel: w1844 -> [w1858 _]
                          disable-tunnel: w1843 -> [w1857 _]
                          disable-tunnel: [w1856 _] -> w1842
                          disable-tunnel: [w1855 _] -> w1838
                          disable-tunnel: w1836 -> [w1854 _]
                          frame Disabled {
                            n350 = call "Stack_holderwise_total_bd_count_&_duration.vi"("Refnum in"=w1860, "BREAKDOWN_STK_HOLD_ID"=3, "condition"=w1854, "Form Date"=w1858, "To Date"=w1857, "error in (no error)"=w1862) -> ("Refnum out"=w1859:T2, "Count out"=w1856:string[], "appended array"=w1855:dbl[], "error out"=w1861:errorcluster)  [unwired: 6 in]
                          }
                          frame Enabled {
                          }
                        }
                        n351 = call "Insert_empty_element_with_zero.vi"("searched date"=w1842, "fixed date"=w1839) -> ("O/P"=w1841:string[])  [unwired: 9 in]
                        n352 = call "NUMERIC TO STRING.vi"("appended array"=w1838) -> ("Array"=w1837:string[])  [unwired: 4 in]
                        n353 = call "Insert_empty_element_with_zero.vi"("searched date"=w1837, "fixed date"=w1839) -> ("O/P"=w1840:string[])  [unwired: 9 in]
                      }
                      frame #4 {
                        n354 = disable-structure shown="Enabled" {
                          disable-tunnel: w1879 -> [w1895 w1898]
                          disable-tunnel: w1878 -> [w1894 w1897]
                          disable-tunnel: [w1893 w1897] -> w1877
                          disable-tunnel: [w1892 w1898] -> w1876
                          disable-tunnel: w1875 -> [w1891 _]
                          disable-tunnel: w1874 -> [w1890 _]
                          disable-tunnel: [w1889 _] -> w1873
                          disable-tunnel: [w1888 _] -> w1869
                          disable-tunnel: w1867 -> [w1887 _]
                          frame Disabled {
                            n355 = call "Stack_holderwise_total_bd_count_&_duration.vi"("Refnum in"=w1894, "BREAKDOWN_STK_HOLD_ID"=4, "condition"=w1887, "Form Date"=w1891, "To Date"=w1890, "error in (no error)"=w1895) -> ("Refnum out"=w1893:T2, "Count out"=w1889:string[], "appended array"=w1888:dbl[], "error out"=w1892:errorcluster)  [unwired: 6 in]
                          }
                          frame Enabled {
                          }
                        }
                        n356 = call "Insert_empty_element_with_zero.vi"("searched date"=w1873, "fixed date"=w1870) -> ("O/P"=w1872:string[])  [unwired: 9 in]
                        n357 = call "NUMERIC TO STRING.vi"("appended array"=w1869) -> ("Array"=w1868:string[])  [unwired: 4 in]
                        n358 = call "Insert_empty_element_with_zero.vi"("searched date"=w1868, "fixed date"=w1870) -> ("O/P"=w1871:string[])  [unwired: 9 in]
                      }
                      frame #5 {
                        n359 = disable-structure shown="Enabled" {
                          disable-tunnel: w1912 -> [w1930 w1933]
                          disable-tunnel: [w1929 w1933] -> w1911
                          disable-tunnel: w1910 -> [w1928 w1932]
                          disable-tunnel: [w1927 w1932] -> w1909
                          disable-tunnel: w1908 -> [w1926 _]
                          disable-tunnel: w1907 -> [w1925 _]
                          disable-tunnel: [w1924 _] -> w1906
                          disable-tunnel: [w1923 _] -> w1902
                          disable-tunnel: w1900 -> [w1922 _]
                          frame Disabled {
                            n360 = call "Stack_holderwise_total_bd_count_&_duration.vi"("Refnum in"=w1928, "BREAKDOWN_STK_HOLD_ID"=5, "condition"=w1922, "Form Date"=w1925, "To Date"=w1926, "error in (no error)"=w1930) -> ("Refnum out"=w1927:T2, "Count out"=w1924:string[], "appended array"=w1923:dbl[], "error out"=w1929:errorcluster)  [unwired: 6 in]
                          }
                          frame Enabled {
                          }
                        }
                        n361 = call "NUMERIC TO STRING.vi"("appended array"=w1902) -> ("Array"=w1901:string[])  [unwired: 4 in]
                        n362 = call "Insert_empty_element_with_zero.vi"("searched date"=w1906, "fixed date"=w1904) -> ("O/P"=w1905:string[])  [unwired: 9 in]
                        n363 = call "Insert_empty_element_with_zero.vi"("searched date"=w1901, "fixed date"=w1904) -> ("O/P"=w1903:string[])  [unwired: 9 in]
                      }
                      frame #6 {
                        n364 = call "String to numeric.vi"("Array"=w1944) -> ("Array 2"=w1943:dbl[])  [unwired: 4 in]
                        n365 = call "String to numeric.vi"("Array"=w1942) -> ("Array 2"=w1941:dbl[])  [unwired: 4 in]
                        n366 = call "String to numeric.vi"("Array"=w1940) -> ("Array 2"=w1939:dbl[])  [unwired: 4 in]
                        n367 = call "String to numeric.vi"("Array"=w1938) -> ("Array 2"=w1937:dbl[])  [unwired: 4 in]
                        n368 = call "String to numeric.vi"("Array"=w1936) -> ("Array 2"=w1935:dbl[])  [unwired: 4 in]
                        n369 = Decimal String To Number(string=w1949) -> (number=w1968:i32[])  [unwired: 2 in, 1 out]
                        n370 = Decimal String To Number(string=w1950) -> (number=w1969:i32[])  [unwired: 2 in, 1 out]
                        n371 = Decimal String To Number(string=w1951) -> (number=w1970:i32[])  [unwired: 2 in, 1 out]
                        n372 = Decimal String To Number(string=w1952) -> (number=w1971:i32[])  [unwired: 2 in, 1 out]
                        n373 = Decimal String To Number(string=w1953) -> (number=w1966:i32[])  [unwired: 2 in, 1 out]
                        n374 = Compound Arithmetic op=ADD(w1943, w1941, w1939, w1937, w1935) -> (w1946:dbl[])
                        n375 = Build Array(w1944) -> (w1965:string[][])
                        n376 = Build Array(w1942) -> (w1964:string[][])
                        n377 = Build Array(w1940) -> (w1963:string[][])
                        n378 = Build Array(w1938) -> (w1962:string[][])
                        n379 = Build Array(w1936) -> (w1961:string[][])
                        n380 = Number To Fractional String(number=w1946, precision (6)=i16 2) -> (F-format string=w1945:string[])  [unwired: 2 in]
                        n381 = Compound Arithmetic op=ADD(w1968, w1969, w1970, w1971, w1966) -> (w1972:i32[])
                        n382 = Transpose 2D Array(2D array=w1965) -> (transposed array=w1959:string[][])
                        n383 = Transpose 2D Array(2D array=w1964) -> (transposed array=w1958:string[][])
                        n384 = Transpose 2D Array(2D array=w1963) -> (transposed array=w1957:string[][])
                        n385 = Transpose 2D Array(2D array=w1962) -> (transposed array=w1956:string[][])
                        n386 = Transpose 2D Array(2D array=w1961) -> (transposed array=w1955:string[][])
                        n387 = Number To Decimal String(number=w1972) -> (decimal integer string=w1967:string[])  [unwired: 1 in]
                        n388 = Build Array(w1945) -> (w1948:string[][])
                        n389 = Transpose 2D Array(2D array=w1948) -> (transposed array=w1954:string[][])
                      }
                      frame #7 {
                        w1975 = string[] ["0"]
                        n390 = Insert Into Array(array=w1985, index (col)=1 ("disabled index (col)"), new element #1=w1984, new element #2=w1983, new element #3=w1975, new element #4=w1975, new element #5=w1975, new element #6=w1975, new element #7=w1975, new element #8=w1975, new element #9=w1975, new element #10=w1975, new element #11=w1976, new element #12=w1977) -> (w1979:string[][])  [unwired: 1 in]
                        n391 = call "flot graph for month n year.vi"("BD Date"=w1980, "error in (no error)"=w1982, "Count total"=w1976) -> ("error out"=w1981:errorcluster, "Run-Time Status"=w1978:cluster{"Array 2":timestamp[], dbl[]})  [unwired: 7 in]
                        n392 = local write "Run-Time Status"(w1978) -> ()
                        n393 = local write "Table"(w1979) -> ()
                      }
                    }
                  }
                  frame "1" {
                    n394 = flat-sequence {
                      tunnel: w1996 -> [w2110]
                      tunnel: w1995 -> [w2108]
                      tunnel: [w2094] -> w2086
                      tunnel: [w2109] -> w2085
                      tunnel: w1994 -> [_]
                      tunnel: [w2113] -> w2084
                      tunnel: [w2093] -> w2083
                      tunnel: [w2092] -> w2082
                      tunnel: [w2091] -> w2081
                      tunnel: w1993 -> [w2093]
                      tunnel: w1992 -> [w2092]
                      tunnel: ["Where BREAKDOWN_DATE between '%s'and '%s' and BREAKDOWN_STK_HOLD_ID ='%d' and  SHIFT_ID = '%d' "] -> w2080
                      tunnel: [w2091] -> w2079
                      tunnel: w1991 -> [w2087]
                      tunnel: [w2087] -> w1990
                      tunnel: w2086 -> [w2174]
                      tunnel: w2085 -> [w2176]
                      tunnel: w2084 -> [w2171]
                      tunnel: w2083 -> [w2170]
                      tunnel: w2082 -> [w2169]
                      tunnel: [w2173] -> w2078
                      tunnel: [w2175] -> w2077
                      tunnel: [w2171] -> w2076
                      tunnel: [w2161] -> w2075
                      tunnel: [w2167] -> w2074
                      tunnel: [w2170] -> w2073
                      tunnel: [w2169] -> w2072
                      tunnel: w2081 -> [w2166]
                      tunnel: [w2166] -> w2071
                      tunnel: w2080 -> [w2163]
                      tunnel: [w2163] -> w2070
                      tunnel: [w2162] -> w2069
                      tunnel: w2079 -> [w2162]
                      tunnel: w1990 -> [w2160]
                      tunnel: w2078 -> [w2190]
                      tunnel: w2077 -> [w2188]
                      tunnel: w2076 -> [w2193]
                      tunnel: w2075 -> [w2192]
                      tunnel: w2074 -> [w2191]
                      tunnel: w2073 -> [w2186]
                      tunnel: w2072 -> [w2185]
                      tunnel: [w2193] -> w2068
                      tunnel: [w2192] -> w2067
                      tunnel: [w2191] -> w2066
                      tunnel: [w2189] -> w2065
                      tunnel: [w2183] -> w2064
                      tunnel: [w2182] -> w2063
                      tunnel: [w2187] -> w2062
                      tunnel: [w2186] -> w2061
                      tunnel: [w2185] -> w2060
                      tunnel: w2071 -> [w2181]
                      tunnel: [w2181] -> w2059
                      tunnel: w2070 -> [w2178]
                      tunnel: [w2178] -> w2058
                      tunnel: [w2177] -> w2057
                      tunnel: w2069 -> [w2177]
                      tunnel: w2068 -> [w2224]
                      tunnel: w2067 -> [w2223]
                      tunnel: w2066 -> [w2222]
                      tunnel: w2065 -> [w2219]
                      tunnel: w2064 -> [w2221]
                      tunnel: w2063 -> [w2220]
                      tunnel: w2062 -> [w2217]
                      tunnel: w2061 -> [w2215]
                      tunnel: w2060 -> [w2214]
                      tunnel: [w2224] -> w2056
                      tunnel: [w2223] -> w2055
                      tunnel: [w2222] -> w2054
                      tunnel: [w2221] -> w2053
                      tunnel: [w2220] -> w2052
                      tunnel: [w2218] -> w2051
                      tunnel: [w2212] -> w2050
                      tunnel: [w2211] -> w2049
                      tunnel: [w2216] -> w2048
                      tunnel: [w2215] -> w2047
                      tunnel: [w2214] -> w2046
                      tunnel: w2059 -> [w2210]
                      tunnel: [w2210] -> w2045
                      tunnel: w2058 -> [w2207]
                      tunnel: [w2207] -> w2044
                      tunnel: [w2206] -> w2043
                      tunnel: w2057 -> [w2206]
                      tunnel: w2056 -> [w2257]
                      tunnel: w2055 -> [w2256]
                      tunnel: w2054 -> [w2255]
                      tunnel: w2053 -> [w2254]
                      tunnel: w2052 -> [w2253]
                      tunnel: w2051 -> [w2250]
                      tunnel: w2050 -> [w2252]
                      tunnel: w2049 -> [w2251]
                      tunnel: w2048 -> [w2249]
                      tunnel: w2047 -> [w2246]
                      tunnel: w2046 -> [w2245]
                      tunnel: [w2257] -> w2042
                      tunnel: [w2256] -> w2041
                      tunnel: [w2255] -> w2040
                      tunnel: [w2254] -> w2039
                      tunnel: [w2253] -> w2038
                      tunnel: [w2252] -> w2037
                      tunnel: [w2251] -> w2036
                      tunnel: [w2248] -> w2035
                      tunnel: [w2247] -> w2034
                      tunnel: [w2243] -> w2033
                      tunnel: [w2242] -> w2032
                      tunnel: [w2246] -> w2031
                      tunnel: [w2245] -> w2030
                      tunnel: w2045 -> [w2241]
                      tunnel: [w2241] -> w2029
                      tunnel: w2044 -> [w2238]
                      tunnel: [w2238] -> w2028
                      tunnel: [w2237] -> w2027
                      tunnel: w2043 -> [w2237]
                      tunnel: w2042 -> [w2292]
                      tunnel: w2041 -> [w2291]
                      tunnel: w2040 -> [w2290]
                      tunnel: w2039 -> [w2289]
                      tunnel: w2038 -> [w2288]
                      tunnel: w2037 -> [w2287]
                      tunnel: w2036 -> [w2286]
                      tunnel: w2035 -> [w2281]
                      tunnel: w2034 -> [w2283]
                      tunnel: w2033 -> [w2285]
                      tunnel: w2032 -> [w2284]
                      tunnel: w2031 -> [w2278]
                      tunnel: w2030 -> [w2279]
                      tunnel: [w2292] -> w2026
                      tunnel: [w2291] -> w2025
                      tunnel: [w2290] -> w2024
                      tunnel: [w2289] -> w2023
                      tunnel: [w2288] -> w2022
                      tunnel: [w2287] -> w2021
                      tunnel: [w2286] -> w2020
                      tunnel: [w2285] -> w2019
                      tunnel: [w2284] -> w2018
                      tunnel: [w2282] -> w2017
                      tunnel: [w2280] -> w2016
                      tunnel: [w2276] -> w2015
                      tunnel: [w2274] -> w2014
                      tunnel: w2029 -> [w2275]
                      tunnel: w2028 -> [w2271]
                      tunnel: [w2270] -> w2013
                      tunnel: w2027 -> [w2270]
                      tunnel: w2026 -> [w2331]
                      tunnel: w2025 -> [w2324]
                      tunnel: w2024 -> [w2315]
                      tunnel: w2023 -> [w2323]
                      tunnel: w2022 -> [w2313]
                      tunnel: w2021 -> [w2322]
                      tunnel: w2020 -> [w2311]
                      tunnel: w2019 -> [w2321]
                      tunnel: w2018 -> [w2309]
                      tunnel: w2017 -> [w2345]
                      tunnel: w2016 -> [w2344]
                      tunnel: w2015 -> [w2320]
                      tunnel: w2014 -> [w2307]
                      tunnel: [w2345] -> w2012
                      tunnel: [w2344] -> w2011
                      tunnel: [w2338] -> w2010
                      tunnel: [w2331] -> w2009
                      tunnel: [w2330] -> w2008
                      tunnel: [w2329] -> w2007
                      tunnel: [w2328] -> w2006
                      tunnel: [w2327] -> w2005
                      tunnel: [w2326] -> w2004
                      tunnel: [w2325] -> w2003
                      tunnel: [w2324] -> w2002
                      tunnel: [w2323] -> w2001
                      tunnel: [w2322] -> w2000
                      tunnel: [w2321] -> w1999
                      tunnel: [w2320] -> w1998
                      tunnel: [w2305] -> w1997
                      tunnel: w2013 -> [w2305]
                      tunnel: [w2358] -> w1988
                      tunnel: [w2352] -> w1989
                      tunnel: w2012 -> [w2353]
                      tunnel: w2011 -> [w2358]
                      tunnel: w2010 -> [w2347]
                      tunnel: w2009 -> [w2356]
                      tunnel: w2008 -> [w2354]
                      tunnel: w2007 -> [_]
                      tunnel: w2006 -> [_]
                      tunnel: w2005 -> [_]
                      tunnel: w2004 -> [_]
                      tunnel: w2003 -> [w2348]
                      tunnel: w2002 -> [w2355]
                      tunnel: w2001 -> [_]
                      tunnel: w2000 -> [_]
                      tunnel: w1999 -> [_]
                      tunnel: w1998 -> [_]
                      tunnel: w1997 -> [w2351]
                      frame #0 {
                        w2101 = "%Y-%m-%d" ("time format string (%c)")
                        n395 = Decimal String To Number(string=w2087) -> (number=w2088:i32)  [unwired: 2 in, 1 out]
                        n396 = property on="Table" class="Tbl (strict)"("Visible"=TRUE) -> ()  [unwired: 2 in, 2 out]
                        n397 = Format Date/Time String(time format string (%c)=w2101, seconds (now)=w2093) -> (date/time string=w2102:string)  [unwired: 1 in]
                        n398 = Format Date/Time String(time format string (%c)=w2101, seconds (now)=w2092) -> (date/time string=w2100:string)  [unwired: 1 in]
